vi "observacao.vi"() -> ()   [LabVIEW 2012] (continued)
          frame True {
            n1066 = local write "Setup, Pointing & Guiding"(T2."ROTATOR" ("Setup, Pointing & Guiding")) -> ()
          }
        }
      }
      frame #2 {
        n1067 = case shown="\"UTILS \"" "Setup, Pointing & Guiding" {
          frame "POINTING", Default {
            n1068 = stacked-sequence {
              frame #0 {
                # "Clear Dados"
                n1069 = case shown="True" "BtPointObjClear" {
                  frame False {
                  }
                  frame True {
                    w1385 = ""
                    n1070 = local write "StrPointObjName"(w1385) -> ()
                    n1071 = local write "StrPointObjPMRA"(w1385) -> ()
                    n1072 = local write "StrPointObjPMDEC"(w1385) -> ()
                    n1073 = local write "StrPointObjRA"(w1385) -> ()
                    n1074 = local write "StrPointObjDEC"(w1385) -> ()
                    n1075 = local write "StrPointObjEpoch"(w1385) -> ()
                    n1076 = local write "StrPointTargetRA"(w1385) -> ()
                    n1077 = local write "StrPointTargetDEC"(w1385) -> ()
                  }
                }
                n1078 = local read "ChkCalLocal"() -> (w1382:bool)
                n1079 = case shown="False" w1382 {
                  selector: w1382 -> [w1384 _]
                  frame False {
                    # "Para de Piscar/Blink\no botão"
                    n1080 = property on="ChkCalLocal" class="Bool (strict)"("Blinking"=w1384) -> ()  [unwired: 2 in, 2 out]
                  }
                  frame True {
                  }
                }
              }
              frame #1 {
                w1392 = ""
                # "A forma como os mostradores da janela TARGET são carregados está indefinida.\nVamos colocar um botão SET ao lado do botão CLEAR na janela OBJECT.\nQuando o botão SET for pressionado, os mostradores da janela TARGET\nseriam calculados a partir dos valores da janela OBJECT."
                n1081 = local read "StrPointObjDEC"() -> (w1393:string)
                n1082 = local read "StrPointObjRA"() -> (w1394:string)
                n1083 = local read "StrPointObjPMDEC"() -> (w1386:string)
                n1084 = local read "StrPointObjPMRA"() -> (w1387:string)
                n1085 = Not Equal?(x=w1394, y=w1392) -> (x != y?=w1391:bool)
                n1086 = Not Equal?(x=w1393, y=w1392) -> (x != y?=w1390:bool)
                n1087 = local read "pressão atm"() -> (w1396:string)
                n1088 = local read "Temp amb"() -> (w1397:string)
                n1089 = local read "hum local"() -> (w1395:string)
                n1090 = And(x=w1391, y=w1390) -> (x .and. y?=w1388:bool)
                n1091 = And(x="BtPointPrecess", y=w1388) -> (x .and. y?=w1389:bool)
                n1092 = case shown="True" w1389 {
                  tunnel: w1394 -> [_ w1405]
                  tunnel: w1393 -> [_ w1404]
                  tunnel: w1397 -> [_ w1403]
                  tunnel: w1396 -> [_ w1402]
                  tunnel: w1395 -> [_ w1401]
                  tunnel: w1387 -> [_ w1400]
                  tunnel: w1386 -> [_ w1399]
                  frame False {
                  }
                  frame True {
                    n1093 = stacked-sequence {
                      tunnel: w1405 -> [w1439 _ _]
                      tunnel: w1404 -> [w1437 _ _]
                      tunnel: w1403 -> [w1447 _ _]
                      tunnel: w1402 -> [w1446 _ _]
                      tunnel: w1401 -> [w1445 _ _]
                      tunnel: w1400 -> [w1413 _ _]
                      tunnel: w1399 -> [w1412 _ _]
                      frame #0 {
                        # "PROCESSO PRECESSÃO"
                        # "MUDANÇA:\nVI Botao SET trocada por Botao Precess, eliminando entrada do Frame de coord. (Mean, Topo, Geo)"
                        n1094 = local read "ChkPointPrecessed"() -> (w1417:bool)
                        n1095 = call "Comma_to_Point.vi"("Lat_A"=w1445) -> ("Saída"=w1414:string)
                        n1096 = call "Comma_to_Point.vi"("Lat_A"=w1447) -> ("Saída"=w1416:string)
                        n1097 = call "Comma_to_Point.vi"("Lat_A"=w1446) -> ("Saída"=w1415:string)
                        n1098 = call "Comma_to_Point.vi"("Lat_A"=w1437) -> ("Saída"=w1432:string)
                        n1099 = call "Comma_to_Point.vi"("Lat_A"=w1439) -> ("Saída"=w1435:string)
                        n1100 = call "hms_rad.vi"("True = hora"=FALSE, "Texto Graus"=w1432) -> ("radianos"=w1431:dbl)  [unwired: 3 in]
                        n1101 = call "hms_rad.vi"("True = hora"=TRUE, "Texto Graus"=w1435) -> ("radianos"=w1434:dbl)  [unwired: 3 in]
                        n1102 = call "Arcsec to Rad_ String.vi"("VAR ARCSEC"=w1413) -> ("VAR RAD"=w1411:string)
                        n1103 = Number To Fractional String(use system decimal point (T)=FALSE, number=w1431, precision (6)=i16 9) -> (F-format string=w1420:string)  [unwired: 1 in]
                        n1104 = Number To Fractional String(use system decimal point (T)=FALSE, number=w1434, precision (6)=i16 9) -> (F-format string=w1421:string)  [unwired: 1 in]
                        n1105 = call "Arcsec to Rad_ String.vi"("VAR ARCSEC"=w1412) -> ("VAR RAD"=w1410:string)
                        n1106 = call "Botão Precess.vi"("AR"=w1421, "Precessed Coord."=w1417, "Dec"=w1420, "Temp local amb(K)"=w1416, "Pressao atm local (mB)"=w1415, "Hum rel local"=w1414, "Var RA"=w1411, "Var DEC"=w1410) -> ("RA"=w1449:dbl, "DEC"=w1406:dbl, "Hora Sideral (rad)"=w1448:dbl, "Dist. Zenital (rad)"=w1419:dbl, "Observed HA (radians)"=→"HA obs":dbl, "Massa de Ar"=w1418:dbl)  [unwired: 2 in]
                        "RA obs" <- w1449
                        "DEC obs" <- w1406
                        n1107 = local write "Zenital angle"(w1419) -> ()
                        n1108 = call "rad_hms.vi"("TRUE=HORA\nFALSE=GRAU"=FALSE ("TRUE=HORA\nFALSE=GRAU"), "Radiano"=w1406) -> ("Hora/Graus Texto Decimal"=w1427:string)  [unwired: 3 in]
                        n1109 = call "rad-graus.vi"("Radiano"=w1419) -> ("Graus"=w1444:dbl)
                        n1110 = Number To Fractional String(number=w1418, precision (6)=i16 3) -> (F-format string=→"Air Mass":string)  [unwired: 2 in]
                        n1111 = Number To Fractional String(number=w1444, precision (6)=i16 1) -> (F-format string=→"Zenital Angle":string)  [unwired: 2 in]
                        n1112 = call "rad_hms.vi"("TRUE=HORA\nFALSE=GRAU"=TRUE ("TRUE=HORA"), "Radiano"=w1449) -> ("Hora/Graus Texto Decimal"=w1429:string)  [unwired: 3 in]
                        n1113 = local write "StrPointTargetDEC"(w1427) -> ()
                        n1114 = local write "StrPointTargetRA"(w1429) -> ()
                        n1115 = disable-structure shown="Disabled" {
                          disable-tunnel: [w1453 _] -> _
                          disable-tunnel: w1449 -> [w1452 _]
                          disable-tunnel: w1448 -> [w1451 _]
                          disable-tunnel: w1406 -> [w1450 _]
                          frame Disabled {
                            n1116 = call "Hora_Limite.vi"("Asc Reta RA rad"=w1452, "Sideral Time rad"=w1451, "Declinação rad"=w1450) -> ("TO Tempo de Observação Horas"=w1453:dbl)  [unwired: 2 in]
                          }
                          frame Enabled {
                          }
                        }
                        n1117 = call "Novo_tempo_obs_inicial.vi"("TS"=w1448, "RA"=w1449, "DEC"=w1406) -> ("TO rad"=w1407:dbl)  [unwired: 7 in, 1 out]
                        n1118 = case shown="True" "TRUE=HORA\nFALSE=GRAU" {
                          frame False {
                          }
                          frame True {
                            # "Sincroniza hora do\nPC com GPS"
                            n1119 = call "About_Time.vi"() -> ()  [unwired: 1 in]
                          }
                        }
                        n1120 = call "rad_hms.vi"("TRUE=HORA\nFALSE=GRAU"=TRUE ("TRUE=HORA\nFALSE=GRAU"), "Radiano"=w1407) -> ("Hora/Graus Texto Decimal"=→"Tempo Obs":string)  [unwired: 3 in]
                      }
                      frame #1 {
                        # "Testa o ângulo zenital menor que 70º o led \"Working Area\" \naceso na cor verde se o ângulozenital menor que 70º e \nvermelho em caso cont rário."
                        n1121 = global read "Global_Telescopio.vi" "Piscar working area"() -> (w1460:bool)
                        n1122 = global read "Global_Telescopio.vi" "working area = VERDE"() -> (w1459:bool)
                        n1123 = global read "Global_Telescopio.vi" "ativar botão GO"() -> (w1457:bool)
                        n1124 = case shown="True" w1459 {
                          frame False {
                            # "False=Vermelho"
                            n1125 = local write "LedPointWorkArea"(FALSE ("LedPointWorkArea")) -> ()
                          }
                          frame True {
                            # "True=Verde"
                            "LedPointWorkArea" <- TRUE ("LedPointWorkArea")
                          }
                        }
                        n1126 = global write "Global_Telescopio.vi" "Botão GO = STOP"(FALSE ("Botão GO = STOP")) -> ()
                        n1127 = case shown="True" w1457 {
                          selector: w1457 -> [_ w1461]
                          frame False {
                          }
                          frame True {
                            n1128 = property on="BtTargetPoint" class="Bool"("Visible"=w1461) -> ()  [unwired: 2 in, 2 out]
                          }
                        }
                        n1129 = global write "Global_Telescopio.vi" "Piscar working area"(w1460) -> ()
                        n1130 = global read "Global_Telescopio.vi" "desativar botão GO"() -> (w1458:bool)
                        n1131 = case shown="True" w1458 {
                          selector: w1458 -> [_ w1463]
                          frame False {
                          }
                          frame True {
                            n1132 = Not(x=w1463) -> (.not. x?=w1462:bool)
                            n1133 = property on="BtTargetPoint" class="Bool"("Visible"=w1462) -> ()  [unwired: 2 in, 2 out]
                          }
                        }
                        n1134 = property on="LedPointWorkArea" class="Bool (strict)"("Visible"=TRUE ("Botão GO = STOP")) -> ()  [unwired: 2 in, 2 out]
                        n1135 = property on="LedPointing" class="Bool (strict)"("Visible"=FALSE) -> ()  [unwired: 2 in, 2 out]
                      }
                      frame #2 {
                        n1136 = global read "Global_Telescopio.vi" "CalDEC Local"() -> (w1471:dbl)
                        n1137 = global read "Global_Telescopio.vi" "CalAH Local"() -> (w1472:dbl)
                        n1138 = local read "ChkCalLocal"() -> (w1466:bool)
                        n1139 = Not Equal To 0?(x=w1472) -> (x != 0?=w1469:bool)
                        n1140 = Not Equal To 0?(x=w1471) -> (x != 0?=w1470:bool)
                        n1141 = Or(x=w1469, y=w1470) -> (x .or. y?=w1467:bool)
                        n1142 = And(x=w1466, y=w1467) -> (x .and. y?=w1468:bool)
                        n1143 = case shown="True" w1468 {
                          frame False {
                          }
                          frame True {
                            n1144 = local read "HA obs"() -> (w1492:dbl)
                            n1145 = local read "DEC obs"() -> (w1486:dbl)
                            n1146 = global read "Global_Telescopio.vi" "AH Zero Local"() -> (w1490:dbl)
                            n1147 = global read "Global_Telescopio.vi" "DEC Zero Local"() -> (w1485:dbl)
                            n1148 = global read "Global_Telescopio.vi" "Raio Máximo"() -> (w1474:dbl)
                            n1149 = Cosine(x=w1486) -> (cos(x)=w1491:dbl)
                            n1150 = Cosine(x=w1485) -> (cos(x)=w1489:dbl)
                            n1151 = Multiply(x=w1492, y=w1491) -> (x*y=w1488:dbl)
                            n1152 = Multiply(x=w1490, y=w1489) -> (x*y=w1487:dbl)
                            n1153 = Subtract(x=w1486, y=w1485) -> (x-y=w1481:dbl)
                            n1154 = Multiply(x=w1481, y=w1481) -> (x*y=w1484:dbl)
                            n1155 = Subtract(x=w1488, y=w1487) -> (x-y=w1480:dbl)
                            n1156 = Multiply(x=w1480, y=w1480) -> (x*y=w1482:dbl)
                            n1157 = Add(x=w1482, y=w1484) -> (x+y=w1483:dbl)
                            n1158 = Square Root(x=w1483) -> (sqrt(x)=w1479:dbl)
                            n1159 = Multiply(x=w1479, y=180.0) -> (x*y=w1477:dbl)
                            n1160 = Divide(x=w1477, y=3.141592653589793) -> (x/y=w1475:dbl)
                            n1161 = Greater?(x=w1475, y=w1474) -> (0:w1473:bool)
                            n1162 = property on="ChkCalLocal" class="Bool (strict)"("Blinking"=w1473) -> ()  [unwired: 2 in, 2 out]
                          }
                        }
                      }
                    }
                  }
                }
              }
              frame #2 {
                # "Clicando-se essa Tecla\nInicia-se o Apontamento"
                n1163 = local read "StrPointObjRA"() -> (w1503:string)
                n1164 = local read "StrPointObjDEC"() -> (w1502:string)
                n1165 = local read "StrPointObjPMDEC"() -> (w1494:string)
                n1166 = local read "pressão atm"() -> (w1495:string)
                n1167 = local read "hum local"() -> (w1501:string)
                n1168 = local read "StrPointObjPMRA"() -> (w1493:string)
                n1169 = local read "Temp amb"() -> (w1496:string)
                n1170 = control-ref of="BtTargetPoint"() -> (w1498:refnum<vi>)
                n1171 = property class="Bool"(reference=w1498) -> ("Boolean Text.Text"=w1499:string)  [unwired: 1 in, 2 out]
                n1172 = Equal?(x=w1499, y="POINT") -> (x = y?=w1497:bool)
                n1173 = case shown="True" "BtTargetPoint" {
                  tunnel: w1503 -> [_ w1509]
                  tunnel: w1502 -> [_ w1513]
                  tunnel: w1496 -> [_ w1510]
                  tunnel: w1495 -> [_ w1511]
                  tunnel: w1501 -> [_ w1512]
                  tunnel: w1497 -> [_ w1507]
                  tunnel: w1494 -> [_ w1506]
                  tunnel: w1493 -> [_ w1505]
                  frame False {
                  }
                  frame True {
                    n1174 = case shown="True" w1507 {
                      selector: w1507 -> [w1515 _]
                      tunnel: w1513 -> [_ w1545]
                      tunnel: w1512 -> [_ w1525]
                      tunnel: w1511 -> [_ w1524]
                      tunnel: w1510 -> [_ w1523]
                      tunnel: w1509 -> [_ w1544]
                      tunnel: w1506 -> [_ w1539]
                      tunnel: w1505 -> [_ w1540]
                      frame False {
                        w1516 = 0 ("estado")
                        # "Zera Máquina de Estado\nPelo Botão STOP"
                        n1175 = Not(x=w1515) -> (.not. x?=w1517:bool)
                        n1176 = local write "LedPointing"(w1515) -> ()
                        n1177 = global write "Global_Telescopio.vi" "Botão GO = STOP"(w1517) -> ()
                        n1178 = call "Stop.vi"() -> ()  [unwired: 1 in, 1 out]
                        n1179 = local write "statDEC"(w1516) -> ()
                        n1180 = local write "statAH"(w1516) -> ()
                        n1181 = local write "statCUP"(w1516) -> ()
                        "Flag Stop" <- TRUE ("Flag Stop")
                      }
                      frame True {
                        w1518 = ""
                        w1543 = FALSE ("use system decimal point (T)")
                        n1182 = call "Comma_to_Point.vi"("Lat_A"=w1544) -> ("Saída"=w1533:string)
                        n1183 = call "Comma_to_Point.vi"("Lat_A"=w1545) -> ("Saída"=w1534:string)
                        n1184 = call "Arcsec to Rad_ String.vi"("VAR ARCSEC"=w1540) -> ("VAR RAD"=w1521:string)
                        n1185 = call "hms_rad.vi"("True = hora"=TRUE, "Texto Graus"=w1533) -> ("radianos"=w1548:dbl)  [unwired: 3 in]
                        n1186 = call "hms_rad.vi"("True = hora"=FALSE, "Texto Graus"=w1534) -> ("radianos"=w1546:dbl)  [unwired: 3 in]
                        n1187 = call "Arcsec to Rad_ String.vi"("VAR ARCSEC"=w1539) -> ("VAR RAD"=w1522:string)
                        n1188 = local write "NAME"(w1518) -> ()
                        n1189 = local write "RA"(w1518) -> ()
                        n1190 = local write "DEC"(w1518) -> ()
                        n1191 = Number To Fractional String(use system decimal point (T)=w1543, number=w1548, precision (6)=i16 9) -> (F-format string=w1520:string)  [unwired: 1 in]
                        n1192 = Number To Fractional String(use system decimal point (T)=w1543, number=w1546, precision (6)=i16 9) -> (F-format string=w1519:string)  [unwired: 1 in]
                        n1193 = Concatenate Strings("Apontamento:" ("string"), "RA= " ("string"), w1533, " " ("string"), "DEC= " ("string"), w1534) -> ()  [unwired: 1 out]
                        n1194 = call "PrecessaoCorrigida.vi"("Coordenada do dia"="ChkPointPrecessed", "HabCorrModelo"="ChkModel", "UseLocalZero"="ChkCalLocal", "UseGlobalZero"="ChkCalGlobal", "RA"=w1520, "DEC"=w1519, "MovProprioRA"=w1521, "MovProprioDEC"=w1522, "Temp amb (K)"=w1523, "Press atm (mB)"=w1524, "Humid relat"=w1525) -> ("Estado"=w1528:i32, "RA"=w1527:dbl, "DEC"=w1526:dbl)  [unwired: 2 out]
                        n1195 = Equal To 0?(x=w1528) -> (x = 0?=w1541:bool)
                        n1196 = case shown="False" w1541 {
                          selector: w1541 -> [w1564 _]
                          tunnel: "ChkCalLocal" -> [w1576 _]
                          tunnel: "ChkCalGlobal" -> [w1575 _]
                          tunnel: w1519 -> [w1574 _]
                          tunnel: w1520 -> [w1573 _]
                          tunnel: w1522 -> [w1570 _]
                          tunnel: w1521 -> [w1569 _]
                          tunnel: w1528 -> [w1551 _]
                          tunnel: w1527 -> [w1572 _]
                          tunnel: w1526 -> [w1571 _]
                          tunnel: "ChkPointPrecessed" -> [w1567 _]
                          frame False {
                            w1554 = FALSE ("Coude")
                            w1555 = FALSE ("WeakSel")
                            w1556 = T10."Enabled" ("Disabled")
                            w1557 = TRUE ("MOUNT")
                            w1568 = 0 ("M_AH")
                            w1565 = TRUE
                            # "ABAS DE CONTROLE"
                            # "MUDANÇA:\nIncluído CASE"
                            # "Seta máquinas de\nestado aba ÚTILS"
                            n1197 = global write "Global_Telescopio.vi" "CoordDia"(w1567) -> ()
                            n1198 = global write "Global_Telescopio.vi" "CalGlobal"(w1575) -> ()
                            n1199 = global write "Global_Telescopio.vi" "CalLocal"(w1576) -> ()
                            n1200 = call "Envia LOG.vi"() -> ()  [unwired: 8 in, 2 out]
                            n1201 = global write "Global_Telescopio.vi" "TargetRA"(w1572) -> ()
                            n1202 = global write "Global_Telescopio.vi" "TargetDEC"(w1571) -> ()
                            n1203 = local write "statAH"(w1551) -> ()
                            n1204 = property on="LedPointWorkArea" class="Bool (strict)"("Visible"=FALSE ("Botão GO = STOP")) -> ()  [unwired: 2 in, 2 out]
                            n1205 = local write "statDEC"(w1551) -> ()
                            n1206 = global write "Global_Telescopio.vi" "ObjCentrado"(w1564) -> ()
                            n1207 = local write "RA on Target"(w1564) -> ()
                            n1208 = local write "DEC on Target"(w1564) -> ()
                            n1209 = local write "Dome on Target"(w1564) -> ()
                            n1210 = local read "ChkDomeEnable"() -> (w1563:bool)
                            n1211 = local write "M_AH"(w1568) -> ()
                            n1212 = local write "M_DEC"(w1568) -> ()
                            n1213 = local write "M_CUP"(w1568) -> ()
                            n1214 = case shown="False" w1563 {
                              selector: w1563 -> [w1597 _]
                              tunnel: w1551 -> [_ w1599]
                              tunnel: [0 ("Estado") w1599] -> w1562
                              tunnel: [u8 2 ("Disabled") u8 0 ("Disabled")] -> w1561
                              frame False {
                                n1215 = local write "DOME"(w1597) -> ()
                              }
                              frame True {
                              }
                            }
                            n1216 = Tick Count (ms)() -> (millisecond timer value=w1559:u32)
                            n1217 = Add(x=w1559, y=u32 120000) -> (x+y=w1560:u32)
                            n1218 = local write "Tick Cupula"(w1560) -> ()
                            n1219 = local write "GUIDER"(w1557) -> ()
                            n1220 = local write "MOUNT"(w1557) -> ()
                            n1221 = property on="LedPointing" class="Bool (strict)"("Visible"=w1565) -> ()  [unwired: 2 in, 2 out]
                            n1222 = local write "statCUP"(w1562) -> ()
                            n1223 = property on="DOME" class="Bool (strict)"("Disabled"=w1561) -> ()  [unwired: 2 in, 2 out]
                            n1224 = stacked-sequence {
                              frame #0 {
                                n1225 = local read "StrPointObjName"() -> (w1577:string)
                                n1226 = local read "StrPointObjRA"() -> (w1578:string)
                                n1227 = local read "StrPointObjDEC"() -> (w1579:string)
                                n1228 = global write "Global_Telescopio.vi" "RA AUX"(w1578) -> ()
                                n1229 = global write "Global_Telescopio.vi" "DEC AUX"(w1579) -> ()
                                n1230 = global write "Global_Telescopio.vi" "NAME OBJETO AUX"(w1577) -> ()
                              }
                              frame #1 {
                                w1581 = u16 4 items=["ZERO", "AH", "DEC", "TUBO", "CUP"] ("Controlador")
                                n1231 = call "Monta Comando.vi"("Comando"="DESLIGAR", "Dispositivo"="FLAT_WEAK", "Controlador"=w1581) -> ()  [unwired: 4 in, 3 out]
                              }
                              frame #2 {
                                w1584 = u16 4 items=["ZERO", "AH", "DEC", "TUBO", "CUP"] ("Controlador")
                                n1232 = call "Monta Comando.vi"("Comando"="DESLIGAR", "Dispositivo"="FLAT_LO", "Controlador"=w1584) -> ()  [unwired: 4 in, 3 out]
                              }
                              frame #3 {
                                w1587 = u16 4 items=["ZERO", "AH", "DEC", "TUBO", "CUP"] ("Controlador")
                                n1233 = call "Monta Comando.vi"("Comando"="DESLIGAR", "Dispositivo"="FLAT_HI", "Controlador"=w1587) -> ()  [unwired: 4 in, 3 out]
                              }
                              frame #4 {
                                w1589 = u16 4 items=["ZERO", "AH", "DEC", "TUBO", "CUP"] ("Controlador")
                                n1234 = call "Monta Comando.vi"("Comando"="DESLIGAR", "Dispositivo"="FLAT_COUDE", "Controlador"=w1589) -> ()  [unwired: 4 in, 3 out]
                              }
                              frame #5 {
                                w1592 = u16 4 items=["ZERO", "AH", "DEC", "TUBO", "CUP"] ("Controlador")
                                n1235 = call "Monta Comando.vi"("Comando"="LIGAR", "Dispositivo"="LAMP_CAM", "Controlador"=w1592) -> ()  [unwired: 4 in, 3 out]
                              }
                              frame #6 {
                                n1236 = call "Log_Apontamento.vi"() -> ()  [unwired: 12 in]
                              }
                            }
                            n1237 = local write "WeakSel"(w1555) -> ()
                            n1238 = local write "MediumSel"(w1555) -> ()
                            n1239 = local write "StrongSel"(w1555) -> ()
                            n1240 = local write "CoudeSel"(w1555) -> ()
                            n1241 = local write "Coude"(w1554) -> ()
                            n1242 = local write "Weak"(w1554) -> ()
                            n1243 = local write "Medium"(w1554) -> ()
                            n1244 = local write "Strong"(w1554) -> ()
                            n1245 = local write "DOME"(FALSE ("WeakSel")) -> ()
                            n1246 = property on="Medium" class="Bool (strict)"("Disabled"=w1556) -> ()  [unwired: 2 in, 2 out]
                            n1247 = property on="Strong" class="Bool (strict)"("Disabled"=w1556) -> ()  [unwired: 2 in, 2 out]
                            n1248 = property on="Coude" class="Bool (strict)"("DisabledEnum"=w1556) -> ()  [unwired: 2 in, 2 out]
                            n1249 = property on="Weak" class="Bool (strict)"("Disabled"=w1556) -> ()  [unwired: 2 in, 2 out]
                            "MeanDEC" <- w1574
                            "MeanRA" <- w1573
                            "LedPointing" <- w1565
                            "PM_DEC" <- w1570
                            "PM_RA" <- w1569
                            "Apontou" <- TRUE ("WeakSel")
                          }
                          frame True {
                          }
                        }
                      }
                    }
                    n1250 = property on="Delete Calagem" class="Bool"("Disabled"=u8 0) -> ()  [unwired: 2 in, 2 out]
                  }
                }
              }
              frame #3 {
                # "e o led \"Working Area\" aceso na cor verde se o ângulo\nzenital menor que 70º e vermelho em caso cont rário.\nO botão GO ao ser clicado dispara o apontamento virtual do telescópio. Caso esse\nbotão seja pressionado enquanto o led \"Working Area\" est iver vermelho, este deve\npiscar 3 vezes e nada mais é executado. Caso cont rário, o nome do botão GO passa\npara CANCEL e o led \"Mount in Posit ion\" da janela STATUS INFORMATION deve ser\ndesligado, o que provocará a simulação do apontamento do telescópio (cf. item 4.3) .\nOs valores dos comandos \"Epoch\" , \"RA Proper Mot ion\" e \"DEC Proper Mot ion\" desse\nquadro devem ser ignorados na simulação."
                # "Habilita Cancela"
                # "Habilita Apontamento"
                n1251 = case shown="True" "Case Constant\n(See Context Help) 5" {
                  frame False {
                  }
                  frame True {
                    w1605 = TRUE ("Go aux")
                    w1606 = ""
                    n1252 = local write "LED MOUNT"(w1605) -> ()
                    n1253 = local write "MOUNT"(w1605) -> ()
                    n1254 = control-ref of="BtTargetPoint"() -> (w1607:refnum<vi>)
                    n1255 = local write "DEC"(w1606) -> ()
                    n1256 = local write "RA"(w1606) -> ()
                    n1257 = local write "NAME"(w1606) -> ()
                    n1258 = property class="Bool"(reference=w1607, "Boolean Text.Text"="STOP") -> ()  [unwired: 1 in, 2 out]
                  }
                }
                n1259 = case shown="True" "Case Constant\n(See Context Help) 6" {
                  frame False {
                  }
                  frame True {
                    w1602 = FALSE ("Go aux")
                    # "Seta nome para GO"
                    n1260 = local write "LED MOUNT"(w1602) -> ()
                    n1261 = local write "MOUNT"(w1602) -> ()
                    n1262 = control-ref of="BtTargetPoint"() -> (w1603:refnum<vi>)
                    n1263 = property class="Bool"(reference=w1603, "Boolean Text.Text"="POINT") -> ()  [unwired: 1 in, 2 out]
                  }
                }
              }
              frame #4 {
                # "Detecta Edição"
                # "os valores de RA e DEC devem assumir os valores da janela OBJECT da aba POINTING ao TÉRMINO do apontamento. Durante o apontamento devem ficar apagados. Como o campo MAG daquela janela não tem um valor correspondente na janela OBJECT, o campo MAG deve ficar em branco. Apenas quando as coordenadas da janela OBJECT da aba POINTING forem preenchidos a partir do botão SET COORD da aba LIST é que o campo MAG da janela TARGET assume o valor da coluna MAG da aba LIST. Colocar um flag interno (invisível para o usuário) para definir se o campo MAG deve ou não ser preenchido com o valor da aba LIST. Quando o botão SET COORD. fosse pressionado esse flag assumiria o valor verdadeiro e caso ocorresse edição dos valores da janela \nOBJECT da aba POINTING, esse flag assumiria o valor falso e o campo MAG da janela TARGET (entre os controles das abas e as imagens) ficaria vazio durante e após o apontamento"
                n1264 = local read "StrPointObjPMRA"() -> (w1622:string)
                n1265 = local read "StrPointObjPMDEC"() -> (w1621:string)
                n1266 = local read "StrPointObjName"() -> (w1629:string)
                n1267 = local read "AUX EDITA Name"() -> (w1628:string)
                n1268 = local read "StrPointObjEpoch"() -> (w1623:string)
                n1269 = local read "AUX EDITA PMDEC"() -> (w1620:string)
                n1270 = local read "StrPointObjRA"() -> (w1627:string)
                n1271 = local read "StrPointObjDEC"() -> (w1625:string)
                n1272 = local read "AUX EDITA EPOCH"() -> (w1618:string)
                n1273 = local read "AUX EDITA PMRA"() -> (w1619:string)
                n1274 = local read "AUX EDITA DEC"() -> (w1624:string)
                n1275 = local read "AUX EDITA RA"() -> (w1626:string)
                n1276 = Not Equal?(x=w1622, y=w1619) -> (x != y?=w1613:bool)
                n1277 = Not Equal?(x=w1629, y=w1628) -> (x != y?=w1617:bool)
                n1278 = Not Equal?(x=w1623, y=w1618) -> (x != y?=w1614:bool)
                n1279 = Not Equal?(x=w1621, y=w1620) -> (x != y?=w1612:bool)
                n1280 = Not Equal?(x=w1627, y=w1626) -> (x != y?=w1616:bool)
                n1281 = Not Equal?(x=w1625, y=w1624) -> (x != y?=w1615:bool)
                n1282 = Compound Arithmetic op=OR(w1617, w1616, w1615, w1614, w1613, w1612) -> (w1609:bool)
                n1283 = local read "FLAG SET COORD"() -> (w1610:bool)
                n1284 = And(x=w1609, y=w1610) -> (x .and. y?=w1611:bool)
                n1285 = case shown="True" w1611 {
                  frame False {
                  }
                  frame True {
                    # "Se houver edição o flag é resetado"
                    n1286 = local write "MAG"("") -> ()
                    "FLAG SET COORD" <- FALSE ("FLAG SET ACOORD")
                  }
                }
              }
            }
          }
          frame "HANDSET" {
            # "PROCESSO DISPLAY DESLOCAMENTO"
            n1287 = local read "AtualDEC"() -> (w1645:dbl)
            n1288 = global read "Global_Telescopio.vi" "Sideral Time"() -> (w1638:dbl)
            n1289 = global read "Global_Telescopio.vi" "PosAH"() -> (w1636:dbl)
            n1290 = Multiply(x="Velocity (arcsec/sec)", y=100.0) -> (x*y=w1653:dbl)
            n1291 = Cosine(x=w1645) -> (cos(x)=w1644:dbl)
            n1292 = Subtract(x=w1638, y=w1636) -> (x-y=w1637:dbl)
            n1293 = Absolute Value(x=w1644) -> (abs(x)=w1641:dbl)
            n1294 = Add(x=1e-10, y=w1641) -> (x+y=w1643:dbl)
            n1295 = local read "LatchDeslocRA"() -> (w1649:dbl)
            n1296 = local read "LatchDeslocDEC"() -> (w1648:dbl)
            n1297 = global read "Global_Telescopio.vi" "PosDEC"() -> (w1639:dbl)
            n1298 = event shown="[9] \"Calagem\": Value Change" {
              selector: _ -> [_ _ _ _ _ _ _ _ _ _ _]
              dyn-events: _ -> [_ _ _ _ _ _ _ _ _ _ _]
              timeout: 10 -> [_ _ _ _ _ _ _ _ _ _ _]
              tunnel: w1653 -> [_ w1666 w1674 w1682 _ _ _ _ _ _ w1785]
              tunnel: "Global" -> [_ _ _ _ _ _ _ _ w1727 w1747 _]
              tunnel: w1637 -> [_ _ _ _ w1685 _ _ _ _ w1745 _]
              tunnel: w1639 -> [_ _ _ _ _ w1686 _ _ _ w1746 _]
              tunnel: w1643 -> [_ _ _ _ _ _ w1687 w1705 _ _ _]
              event Timeout {
                n1299 = event-data() -> ()  [unwired: 1 in, 2 out]
              }
              event "Left HS": Value Change {
                w1663 = u8 0 ("Disabled")
                n1300 = event-data() -> ("NewVal"=w1662:bool)  [unwired: 1 in, 5 out]
                "MOV_IDX_AH" <- w1662
                n1301 = Select(t=u8 2 ("Disabled"), s=FALSE, f=w1663) -> (s? t:f=w1664:u8)
                n1302 = call "Tx handeset.vi"("CMD On"="left" ("Comando"), "CMD Off"="stoph" ("Comando"), "Estado do Botão"=w1662, "Velocity (arcsec/sec)"=w1666) -> ()  [unwired: 12 in]
                n1303 = property on="Delete Calagem" class="Bool"("Disabled"=w1663) -> ()  [unwired: 2 in, 2 out]
                n1304 = property on="Right HS" class="Bool (strict)"("Disabled"=w1664) -> ()  [unwired: 2 in, 2 out]
              }
              event "Down HS": Value Change {
                w1670 = u8 0 ("Disabled")
                n1305 = event-data() -> ("NewVal"=w1673:bool)  [unwired: 1 in, 5 out]
                "MOV_IDX_DEC" <- w1673
                n1306 = call "Tx handeset.vi"("CMD On"="down" ("Comando"), "CMD Off"="stopv" ("Comando"), "Estado do Botão"=w1673, "Velocity (arcsec/sec)"=w1674) -> ()  [unwired: 12 in]
                n1307 = Select(t=u8 2 ("Disabled"), s=FALSE, f=w1670) -> (s? t:f=w1671:u8)
                n1308 = property on="Delete Calagem" class="Bool"("Disabled"=w1670) -> ()  [unwired: 2 in, 2 out]
                n1309 = property on="Up HS" class="Bool (strict)"("Disabled"=w1671) -> ()  [unwired: 2 in, 2 out]
              }
              event "Right HS": Value Change {
                w1679 = u8 0 ("Disabled")
                n1310 = event-data() -> ("NewVal"=w1678:bool)  [unwired: 1 in, 5 out]
                n1311 = call "Tx handeset.vi"("CMD On"="right" ("Comando"), "CMD Off"="stoph" ("Comando"), "Estado do Botão"=w1678, "Velocity (arcsec/sec)"=w1682) -> ()  [unwired: 12 in]
                n1312 = Select(t=u8 2 ("Disabled"), s=FALSE, f=w1679) -> (s? t:f=w1680:u8)
                n1313 = property on="Delete Calagem" class="Bool"("Disabled"=w1679) -> ()  [unwired: 2 in, 2 out]
                n1314 = local write "MOV_IDX_AH"(w1678) -> ()
                n1315 = property on="Left HS" class="Bool (strict)"("Disabled"=w1680) -> ()  [unwired: 2 in, 2 out]
              }
              event "ClearDeslocRA": Value Change {
                n1316 = event-data() -> ()  [unwired: 1 in, 6 out]
                "LatchDeslocRA" <- w1685
              }
              event "ClearDeslocDEC": Value Change {
                n1317 = event-data() -> ()  [unwired: 1 in, 6 out]
                "LatchDeslocDEC" <- w1686
              }
              event "BtPrecCentrar": Value Change {
                # "PROCESSO OFFSET"
                n1318 = event-data() -> ()  [unwired: 1 in, 6 out]
                n1319 = stacked-sequence {
                  tunnel: w1687 -> [_ w1696]
                  frame #0 {
                    n1320 = local read "Offset DEC"() -> (w1688:dbl)
                    n1321 = Negate(x=w1688) -> (-x=w1689:dbl)
                    n1322 = Equal To 0?(x=w1688) -> (x = 0?=w1690:bool)
                    n1323 = case shown="False" w1690 {
                      tunnel: w1689 -> [w1691 _]
                      frame False {
                        n1324 = call "Conversao Ms to Hora texto.vi"("TRUE=HORA\nFALSE=GRAU"=FALSE ("TRUE=HORA\nFALSE=GRAU"), "PrecDEC"=w1691) -> ("Hora/Graus Texto Decimal"=w1693:string)
                        n1325 = call "Tx handeset.vi"("CMD On"="goDEC", "Set Point"=w1693, "Estado do Botão"=TRUE ("TRUE=HORA\nFALSE=GRAU")) -> ()  [unwired: 13 in]
                      }
                      frame True {
                      }
                    }
                  }
                  frame #1 {
                    # "PROCESSO MOVE TELESCÓPIO"
                    n1326 = local read "Offset RA"() -> (w1697:dbl)
                    n1327 = Equal To 0?(x=w1697) -> (x = 0?=w1698:bool)
                    n1328 = case shown="False" w1698 {
                      tunnel: w1697 -> [w1700 _]
                      tunnel: w1696 -> [w1699 _]
                      frame False {
                        w1702 = TRUE ("TRUE=HORA\nFALSE=GRAU")
                        # "AH tem sentido\ncontrário de RA"
                        n1329 = Divide(x=w1700, y=w1699) -> (x/y=w1701:dbl)
                        n1330 = call "Conversao Ms to Hora texto.vi"("TRUE=HORA\nFALSE=GRAU"=w1702, "PrecDEC"=w1701) -> ("Hora/Graus Texto Decimal"=w1703:string)
                        n1331 = call "Tx handeset.vi"("CMD On"="goRA", "Set Point"=w1703, "Estado do Botão"=w1702) -> ()  [unwired: 13 in]
                      }
                      frame True {
                      }
                    }
                  }
                }
              }
              event "BtPrecGO": Value Change {
                # "PROCESSO OFFSET"
                n1332 = event-data() -> ("NewVal"=w1707:bool)  [unwired: 1 in, 5 out]
                n1333 = case shown="True" w1707 {
                  tunnel: w1705 -> [_ w1708]
                  frame False {
                  }
                  frame True {
                    # "PROCESSO MOVE TELESCÓPIO"
                    n1334 = stacked-sequence {
                      tunnel: w1708 -> [_ w1716]
                      frame #0 {
                        n1335 = Not Equal To 0?(x="PreciseOffsetDEC") -> (x != 0?=w1710:bool)
                        n1336 = case shown="True" w1710 {
                          tunnel: "PreciseOffsetDEC" -> [_ w1711]
                          frame False {
                          }
                          frame True {
                            n1337 = call "Conversao Ms to Hora texto.vi"("TRUE=HORA\nFALSE=GRAU"=FALSE ("TRUE=HORA\nFALSE=GRAU"), "PrecDEC"=w1711) -> ("Hora/Graus Texto Decimal"=w1713:string)
                            n1338 = call "Tx handeset.vi"("CMD On"="goDEC", "Set Point"=w1713, "Estado do Botão"=TRUE ("TRUE=HORA\nFALSE=GRAU")) -> ()  [unwired: 13 in]
                          }
                        }
                      }
                      frame #1 {
                        n1339 = Not Equal To 0?(x="PreciseOffsetRA") -> (x != 0?=w1719:bool)
                        n1340 = Negate(x="PreciseOffsetRA") -> (-x=w1718:dbl)
                        n1341 = case shown="True" w1719 {
                          tunnel: w1718 -> [_ w1721]
                          tunnel: w1716 -> [_ w1720]
                          frame False {
                          }
                          frame True {
                            n1342 = Divide(x=w1721, y=w1720) -> (x/y=w1722:dbl)
                            n1343 = call "Conversao Ms to Hora texto.vi"("TRUE=HORA\nFALSE=GRAU"=TRUE ("TRUE=HORA\nFALSE=GRAU"), "PrecDEC"=w1722) -> ("Hora/Graus Texto Decimal"=w1724:string)
                            n1344 = call "Tx handeset.vi"("CMD On"="goRA", "Set Point"=w1724, "Estado do Botão"=TRUE ("TRUE=HORA\nFALSE=GRAU")) -> ()  [unwired: 13 in]
                          }
                        }
                      }
                    }
                  }
                }
                n1345 = property on="Delete Calagem" class="Bool"("Disabled"=u8 2) -> ()  [unwired: 2 in, 2 out]
              }
              event "Delete Calagem": Value Change {
                n1346 = event-data() -> ()  [unwired: 1 in, 6 out]
                n1347 = case shown="True" w1727 {
                  tunnel: 0.0 ("Calagem DEC Rel") -> [w1729 w1730]
                  frame False {
                    # "Local"
                    n1348 = global write "Global_Telescopio.vi" "CalAH Local"(w1729) -> ()
                    n1349 = global write "Global_Telescopio.vi" "CalDEC Local"(w1729) -> ()
                  }
                  frame True {
                    # "Global"
                    n1350 = global write "Global_Telescopio.vi" "Calagem AH"(w1730) -> ()
                    n1351 = global write "Global_Telescopio.vi" "Calagem DEC"(w1730) -> ()
                  }
                }
              }
              event "Calagem": Value Change {
                # "PROCESSO CALAGEM"
                n1352 = event-data() -> ()  [unwired: 1 in, 6 out]
                n1353 = local read "ChkModel"() -> (w1736:bool)
                n1354 = local read "Temp amb"() -> (w1740:string)
                n1355 = local read "hum local"() -> (w1742:string)
                n1356 = local read "MeanDEC"() -> (w1733:string)
                n1357 = local read "pressão atm"() -> (w1741:string)
                n1358 = local read "MeanRA"() -> (w1737:string)
                n1359 = local read "PM_RA"() -> (w1738:string)
                n1360 = local read "PM_DEC"() -> (w1739:string)
                n1361 = global read "Global_Telescopio.vi" "CalGlobal"() -> (w1734:bool)
                n1362 = global read "Global_Telescopio.vi" "CalLocal"() -> (w1735:bool)
                n1363 = global read "Global_Telescopio.vi" "CoordDia"() -> (w1732:bool)
                n1364 = call "PrecessaoCorrigida.vi"("Coordenada do dia"=w1732, "HabCorrModelo"=w1736, "UseLocalZero"=w1735, "UseGlobalZero"=w1734, "RA"=w1737, "DEC"=w1733, "MovProprioRA"=w1738, "MovProprioDEC"=w1739, "Temp amb (K)"=w1740, "Press atm (mB)"=w1741, "Humid relat"=w1742) -> ("RA"=w1744:dbl, "DEC"=w1743:dbl, "AH"=w1731:dbl)  [unwired: 2 out]
                n1365 = case shown="True" w1747 {
                  tunnel: w1744 -> [w1757 w1760]
                  tunnel: w1743 -> [w1749 w1762]
                  tunnel: w1746 -> [w1756 w1763]
                  tunnel: w1745 -> [w1758 w1761]
                  tunnel: w1731 -> [w1748 _]
                  frame False {
                    # "Local"
                    n1366 = Subtract(x=w1758, y=w1757) -> (x-y=w1759:dbl)
                    n1367 = Subtract(x=w1756, y=w1749) -> (x-y=w1753:dbl)
                    n1368 = global read "Global_Telescopio.vi" "CalAH Local"() -> (w1752:dbl)
                    n1369 = global read "Global_Telescopio.vi" "CalDEC Local"() -> (w1754:dbl)
                    n1370 = global write "Global_Telescopio.vi" "AH Zero Local"(w1748) -> ()
                    n1371 = global write "Global_Telescopio.vi" "DEC Zero Local"(w1749) -> ()
                    n1372 = Negate(x=w1759) -> (-x=w1755:dbl)
                    n1373 = Add(x=w1755, y=w1752) -> (x+y=w1751:dbl)
                    n1374 = Add(x=w1753, y=w1754) -> (x+y=w1750:dbl)
                    n1375 = global write "Global_Telescopio.vi" "CalAH Local"(w1751) -> ()
                    n1376 = global write "Global_Telescopio.vi" "CalDEC Local"(w1750) -> ()
                  }
                  frame True {
                    # "Global"
                    n1377 = stacked-sequence {
                      tunnel: w1763 -> [w1773 _ _]
                      tunnel: w1762 -> [w1772 _ _]
                      tunnel: w1761 -> [w1768 _ _]
                      tunnel: w1760 -> [w1767 _ _]
                      frame #0 {
                        w1764 = 0.0 ("CalAH Local")
                        n1378 = Subtract(x=w1768, y=w1767) -> (x-y=w1766:dbl)
                        n1379 = Subtract(x=w1773, y=w1772) -> (x-y=w1774:dbl)
                        n1380 = global read "Global_Telescopio.vi" "Calagem AH"() -> (w1771:dbl)
                        n1381 = global read "Global_Telescopio.vi" "Calagem DEC"() -> (w1776:dbl)
                        n1382 = Negate(x=w1766) -> (-x=w1769:dbl)
                        n1383 = local write "Processa Centragem"(TRUE) -> ()
                        n1384 = Add(x=w1769, y=w1771) -> (x+y=w1770:dbl)
                        n1385 = Add(x=w1774, y=w1776) -> (x+y=w1775:dbl)
                        n1386 = global write "Global_Telescopio.vi" "Calagem AH"(w1770) -> ()
                        n1387 = global write "Global_Telescopio.vi" "CalAH Local"(w1764) -> ()
                        n1388 = global write "Global_Telescopio.vi" "CalDEC Local"(w1764) -> ()
                        n1389 = global write "Global_Telescopio.vi" "Calagem DEC"(w1775) -> ()
                      }
                      frame #1 {
                        # "25/10/2012 - Sempre que o usuario faz uma \ncalagem global, o valor da calagem e'  salva \nautomaticamente em GLOBAIS_CALAGEM.DAT"
                        n1390 = call "Salva_Calagem_Global.vi"() -> ()  [unwired: 1 in]
                      }
                      frame #2 {
                        # "Salva no Logo valor \ndo deslocamento da \ncalagem global"
                        n1391 = local read "DeslocDEC"() -> (w1777:dbl)
                        n1392 = local read "DeslocRA"() -> (w1778:dbl)
                        n1393 = call "Log_Calagem.vi"("Desloc DEC"=w1777, "Desloc RA"=w1778, "File Name"="LOG_COMANDOS.TXT") -> ()  [unwired: 3 in]
                      }
                    }
                  }
                }
              }
              event "Up HS": Value Change {
                w1782 = u8 0 ("Disabled")
                n1394 = event-data() -> ("NewVal"=w1781:bool)  [unwired: 1 in, 5 out]
                n1395 = call "Tx handeset.vi"("CMD On"="up" ("Comando"), "CMD Off"="stopv" ("Comando"), "Estado do Botão"=w1781, "Velocity (arcsec/sec)"=w1785) -> ()  [unwired: 12 in]
                n1396 = property on="Delete Calagem" class="Bool"("Disabled"=w1782) -> ()  [unwired: 2 in, 2 out]
                n1397 = Select(t=u8 2 ("Disabled"), s=FALSE, f=w1782) -> (s? t:f=w1783:u8)
                n1398 = local write "MOV_IDX_DEC"(w1781) -> ()
                n1399 = property on="Down HS" class="Bool (strict)"("Disabled"=w1783) -> ()  [unwired: 2 in, 2 out]
              }
            }
            n1400 = Subtract(x=w1637, y=w1649) -> (x-y=w1646:dbl)
            n1401 = Subtract(x=w1639, y=w1648) -> (x-y=w1650:dbl)
            n1402 = Multiply(x=w1646, y=w1643) -> (x*y=w1647:dbl)
            n1403 = global read "Global_Telescopio.vi" "ObjCentrado"() -> (w1640:bool)
            n1404 = call "Rad to Arcsec.vi"("Radiano"=w1647) -> ("Arcsec"=w1633:dbl)
            n1405 = call "Rad to Arcsec.vi"("Radiano"=w1650) -> ("Arcsec"=w1632:dbl)
            n1406 = case shown="False" w1640 {
              tunnel: [w1656 w1658] -> w1635
              tunnel: [w1656 w1659] -> w1634
              tunnel: w1633 -> [_ w1659]
              tunnel: w1632 -> [_ w1658]
              frame False {
                w1656 = 0.0 ("DeslocRA")
                n1407 = property on="Calagem" class="Bool"("Disabled"=u8 2) -> ()  [unwired: 2 in, 2 out]
              }
              frame True {
                n1408 = property on="Calagem" class="Bool"("Disabled"=u8 0) -> ()  [unwired: 2 in, 2 out]
              }
            }
            "DeslocRA" <- w1634
            "DeslocDEC" <- w1635
          }
          frame "GUIDER" {
            w1798 = 1 ("lower limit")
            w1799 = 400 ("upper limit")
            # "PROCESSO VARIABLE TRACKING"
            n1409 = case shown="True" "ClearRA" {
              frame False {
              }
              frame True {
                n1410 = local write "RA  RATE"(0 ("RA  RATE")) -> ()
              }
            }
            n1411 = call "Borda Subida.vi"("Entrada"="VARIABLE \nTRACKING") -> ("Boolean"=w1804:bool)  [unwired: 4 in]
            n1412 = call "Borda.vi"("Entrada"="VARIABLE \nTRACKING") -> ("Boolean"=w1803:bool)  [unwired: 4 in]
            n1413 = case shown="True" w1803 {
              frame False {
              }
              frame True {
                w1859 = "0" ("Set Point")
                w1865 = u16 2 items=["ZERO", "AH", "DEC", "TUBO", "CUP"] ("Controlador")
                w1862 = u16 1 items=["ZERO", "AH", "DEC", "TUBO", "CUP"] ("Controlador")
                # "Enviando ZERO o controlador para o movimento"
                n1414 = call "Monta Comando.vi"("Set Point"=w1859, "Comando"="GIRAR_VEL", "Dispositivo"="EIXO" ("Comando"), "Controlador"=w1862) -> ()  [unwired: 3 in, 3 out]
                n1415 = call "Monta Comando.vi"("Set Point"=w1859, "Comando"="GIRAR_VEL", "Dispositivo"="EIXO" ("Comando"), "Controlador"=w1865) -> ()  [unwired: 3 in, 3 out]
              }
            }
            n1416 = case shown="True" w1804 {
              frame False {
              }
              frame True {
                w1876 = u16 2 items=["ZERO", "AH", "DEC", "TUBO", "CUP"] ("Controlador")
                w1873 = u16 1 items=["ZERO", "AH", "DEC", "TUBO", "CUP"] ("Controlador")
                # "Enviar esses Valores \npara os controladores"
                n1417 = property on="Calagem" class="Bool"("Disabled"=u8 2) -> ()  [unwired: 2 in, 2 out]
                n1418 = Number To Decimal String(number="RA  RATE") -> (decimal integer string=w1869:string)  [unwired: 1 in]
                n1419 = Number To Decimal String(number="DEC RATE") -> (decimal integer string=w1867:string)  [unwired: 1 in]
                n1420 = call "Monta Comando.vi"("Set Point"=w1869, "Comando"="GIRAR_VEL", "Dispositivo"="EIXO" ("Comando"), "Controlador"=w1873) -> ()  [unwired: 3 in, 3 out]
                n1421 = call "Monta Comando.vi"("Set Point"=w1867, "Comando"="GIRAR_VEL", "Dispositivo"="EIXO" ("Comando"), "Controlador"=w1876) -> ()  [unwired: 3 in, 3 out]
              }
            }
            n1422 = case shown="True" "ClearDEC" {
              frame False {
              }
              frame True {
                n1423 = local write "DEC RATE"(0 ("RA  RATE")) -> ()
              }
            }
            n1424 = In Range and Coerce(upper limit=w1799, x="X STAR", lower limit=w1798) -> (In Range?=w1795:bool)  [unwired: 1 out]
            n1425 = In Range and Coerce(upper limit=w1799, x="Y STAR", lower limit=w1798) -> (In Range?=w1796:bool)  [unwired: 1 out]
            n1426 = In Range and Coerce(upper limit=w1799, x="X CENTER", lower limit=w1798) -> (In Range?=w1794:bool)  [unwired: 1 out]
            n1427 = In Range and Coerce(upper limit=w1799, x="Y CENTER", lower limit=w1798) -> (In Range?=w1793:bool)  [unwired: 1 out]
            n1428 = Compound Arithmetic op=AND(w1795, w1796, w1794, w1793, "XY CENTER") -> (w1797:bool)
            n1429 = case shown="True" w1797 {
              tunnel: "X STAR" -> [_ w1840]
              tunnel: "X CENTER" -> [_ w1839]
              tunnel: "Y STAR" -> [_ w1838]
              tunnel: "Y CENTER" -> [_ w1837]
              frame False {
              }
              frame True {
                # "MUDANÇA: IMPLEMENTADO MOV. XY DO GUIDER EM \n20-05-2011, MAS AINDA NÃO FOI TESTADO..."
                # "rad"
                # "Ativa o envio comando de deslocamento ao controlador"
                n1430 = global read "Global_Telescopio.vi" "guide_ang"() -> (w1828:string)
                n1431 = global read "Global_Telescopio.vi" "guide_nor"() -> (w1829:string)
                n1432 = global read "Global_Telescopio.vi" "guide_cas"() -> (w1836:string)
                n1433 = Subtract(x=w1840, y=w1839) -> (x-y=w1834:i32)
                n1434 = Subtract(x=w1838, y=w1837) -> (x-y=w1833:i32)
                n1435 = global read "Global_Telescopio.vi" "guide_esp"() -> (w1831:string)
                n1436 = To Double Precision Float(number=w1834) -> (double precision float=w1811:dbl)
                n1437 = To Double Precision Float(number=w1833) -> (double precision float=w1812:dbl)
                n1438 = Equal?(x=w1836, y="S") -> (x = y?=w1826:bool)
                n1439 = case shown="True" w1826 {
                  tunnel: w1829 -> [_ w1856]
                  tunnel: w1828 -> [_ w1853]
                  tunnel: [w1849 w1850] -> w1825
                  frame False {
                    # "Foco Coudé"
                    n1440 = call "AnguloFenda.vi"() -> ("AngFenda"=w1849:dbl)  [unwired: 3 in]
                  }
                  frame True {
                    # "Foco Cassegrain"
                    n1441 = Fract/Exp String To Number(use system decimal point (T)=FALSE, string=w1856) -> (number=w1851:dbl)  [unwired: 2 in, 1 out]
                    n1442 = Fract/Exp String To Number(use system decimal point (T)=FALSE, string=w1853) -> (number=w1852:dbl)  [unwired: 2 in, 1 out]
                    n1443 = Add(x=w1852, y=w1851) -> (x+y=w1850:dbl)
                  }
                }
                n1444 = Equal?(x=w1831, y="S") -> (x = y?=w1816:bool)
                n1445 = global write "Global_Telescopio.vi" "Correção Guider"("Habilita Movimento") -> ()
                n1446 = Multiply(x=0.01745329252 ("y"), y=w1825) -> (x*y=w1824:dbl)
                n1447 = Cosine(x=w1824) -> (cos(x)=w1813:dbl)
                n1448 = Sine(x=w1824) -> (sin(x)=w1814:dbl)
                n1449 = Multiply(x=w1811, y=w1813) -> (x*y=w1805:dbl)
                n1450 = Multiply(x=w1813, y=w1812) -> (x*y=w1810:dbl)
                n1451 = Multiply(x=w1812, y=w1814) -> (x*y=w1806:dbl)
                n1452 = Multiply(x=w1814, y=w1811) -> (x*y=w1809:dbl)
                n1453 = Subtract(x=w1810, y=w1809) -> (x-y=w1808:dbl)
                n1454 = Add(x=w1806, y=w1805) -> (x+y=w1807:dbl)
                n1455 = Less Than 0?(x=w1808) -> (x < 0?=w1822:bool)
                n1456 = Less Than 0?(x=w1807) -> (x < 0?=w1818:bool)
                n1457 = case shown="True" w1818 {
                  tunnel: w1816 -> [w1842 w1845]
                  tunnel: [w1841 w1846] -> w1815
                  frame False {
                    n1458 = Select(t="W" ("y"), s=w1842, f="E" ("y")) -> (s? t:f=w1841:string)
                  }
                  frame True {
                    n1459 = Select(t="E" ("y"), s=w1845, f="W" ("y")) -> (s? t:f=w1846:string)
                  }
                }
                n1460 = Select(t="S" ("y"), s=w1822, f="N" ("y")) -> (s? t:f=w1821:string)
                n1461 = Absolute Value(x=w1808) -> (abs(x)=w1819:dbl)
                n1462 = Absolute Value(x=w1807) -> (abs(x)=w1817:dbl)
                n1463 = global write "Global_Telescopio.vi" "guide_dir_we"(w1815) -> ()
                n1464 = global write "Global_Telescopio.vi" "guide_dir_ns"(w1821) -> ()
                n1465 = global write "Global_Telescopio.vi" "guide_dec"(w1819) -> ()
                n1466 = global write "Global_Telescopio.vi" "guide_asc"(w1817) -> ()
              }
            }
            "LED VAR TRACKING" <- "VARIABLE \nTRACKING"
          }
          frame "CALIBRATION" {
            # "Alterado dia 23/07/218"
            n1467 = disable-structure shown="Disabled" {
              frame Disabled {
              }
              frame Enabled {
              }
            }
            n1468 = event shown="[4] \"Coude\": Value Change" {
              selector: _ -> [_ _ _ _ _]
              dyn-events: _ -> [_ _ _ _ _]
              timeout: 10 -> [_ _ _ _ _]
              event Timeout {
                n1469 = event-data() -> ()  [unwired: 1 in, 2 out]
              }
              event "Weak": Value Change {
                w1882 = u16 6 items=["Alarme", "Atencao", "Erro", "Ocupado", "TBD", "LCB", "Trapeira", "Paravento", "DomoRap", "DomoCW", "DomoCCW", "TBD", "Em movimento", "TBD"] ("NomeStatus")
                n1470 = event-data() -> ("NewVal"=w1883:bool)  [unwired: 1 in, 5 out]
                n1471 = call "Bit Status CUP.vi"("NomeStatus"=w1882) -> ("StatBit"=w1881:bool)
                n1472 = case shown="False" w1881 {
                  tunnel: w1883 -> [w1890 _]
                  frame False {
                    w1884 = u16 4 items=["ZERO", "AH", "DEC", "TUBO", "CUP"] ("Controlador")
                    n1473 = case shown="True" w1890 {
                      tunnel: [w1891 TRUE ("WeakSel")] -> w1889
                      tunnel: [w1891 FALSE ("MediumSel")] -> w1887
                      tunnel: [0 2] -> w1886
                      tunnel: ["DESLIGAR" ("Comando") "LIGAR" ("Comando")] -> w1888
                      frame False {
                        w1891 = FALSE ("MediumSel")
                      }
                      frame True {
                        n1474 = local write "DOME"(FALSE) -> ()
                        n1475 = local write "StatShutter"("Busy to Close" ("Status")) -> ()
                      }
                    }
                    n1476 = property on="Coude" class="Bool (strict)"("DisabledEnum"=w1886) -> ()  [unwired: 2 in, 2 out]
                    n1477 = property on="WeakSel" class="Bool (strict)"("Value"=w1889) -> ()  [unwired: 2 in, 2 out]
                    n1478 = property on="CoudeSel" class="Bool (strict)"("Value"=w1887) -> ()  [unwired: 2 in, 2 out]
                    n1479 = property on="Strong" class="Bool (strict)"("Disabled"=w1886) -> ()  [unwired: 2 in, 2 out]
                    n1480 = property on="MediumSel" class="Bool (strict)"("Value"=w1887) -> ()  [unwired: 2 in, 2 out]
                    n1481 = property on="StrongSel" class="Bool (strict)"("Value"=w1887) -> ()  [unwired: 2 in, 2 out]
                    n1482 = property on="Medium" class="Bool (strict)"("Disabled"=w1886) -> ()  [unwired: 2 in, 2 out]
                    n1483 = call "Monta Comando.vi"("Comando"=w1888, "Dispositivo"="FLAT_WEAK", "Controlador"=w1884) -> ()  [unwired: 4 in, 3 out]
                  }
                  frame True {
                    w1900 = FALSE ("Weak")
                    n1484 = Get Date/Time In Seconds() -> (seconds since 1Jan1904=w1903:timestamp)
                    n1485 = Add(x=w1903, y=10.0) -> (x+y=w1904:timestamp)
                    n1486 = property on="WeakSel" class="Bool (strict)"("Value"=w1900) -> ()  [unwired: 2 in, 2 out]
                    n1487 = property on="Weak" class="Bool (strict)"("Value"=w1900) -> ()  [unwired: 2 in, 2 out]
                    n1488 = local write "alarm Time"(w1904) -> ()
                    n1489 = property on="Mensage Alarme" class="Str"("Visible"=TRUE) -> ()  [unwired: 2 in, 2 out]
                    n1490 = local write "Flag Alarm"(TRUE ("Flag Alarm")) -> ()
                  }
                }
              }
              event "Medium": Value Change {
                w1907 = u16 6 items=["Alarme", "Atencao", "Erro", "Ocupado", "TBD", "LCB", "Trapeira", "Paravento", "DomoRap", "DomoCW", "DomoCCW", "TBD", "Em movimento", "TBD"] ("NomeStatus")
                n1491 = event-data() -> ("NewVal"=w1908:bool)  [unwired: 1 in, 5 out]
                n1492 = call "Bit Status CUP.vi"("NomeStatus"=w1907) -> ("StatBit"=w1906:bool)
                n1493 = case shown="False" w1906 {
                  tunnel: w1908 -> [w1915 _]
                  frame False {
                    w1910 = u16 4 items=["ZERO", "AH", "DEC", "TUBO", "CUP"] ("Controlador")
                    n1494 = case shown="True" w1915 {
                      tunnel: [0 2] -> w1912
                      tunnel: [w1917 TRUE] -> w1913
                      tunnel: [w1917 FALSE] -> w1911
                      tunnel: ["DESLIGAR" "LIGAR"] -> w1914
                      frame False {
                        w1917 = FALSE
                      }
                      frame True {
                        n1495 = local write "DOME"(FALSE) -> ()
                        n1496 = local write "StatShutter"("Busy to Close" ("Status")) -> ()
                      }
                    }
                    n1497 = property on="Weak" class="Bool (strict)"("Disabled"=w1912) -> ()  [unwired: 2 in, 2 out]
